vi "Shutdown.vi"(8 "error in (no error)":errorcluster, 9 "Wait Timeout [10000 ms]":i32=10000, 10 "Wait For Shutdown (F)":bool, 11 "Actor API in":refnum<class "Actor API.lvclass">) -> (0 "error out":errorcluster)   [LabVIEW 2015, in "Actor API.lvclass"]
uses:
  Actor API.lvclass
  <vilib>/event_ctls.llb/usereventprio.ctl
  Messaging/Message/Message.lvclass
  Messaging/Message/Message.lvclass/Message.ctl
  Utility/Error Code.ctl
panel:
  # "Note this VI is reentrant as it is called in parallel when shutting down the Top Level"
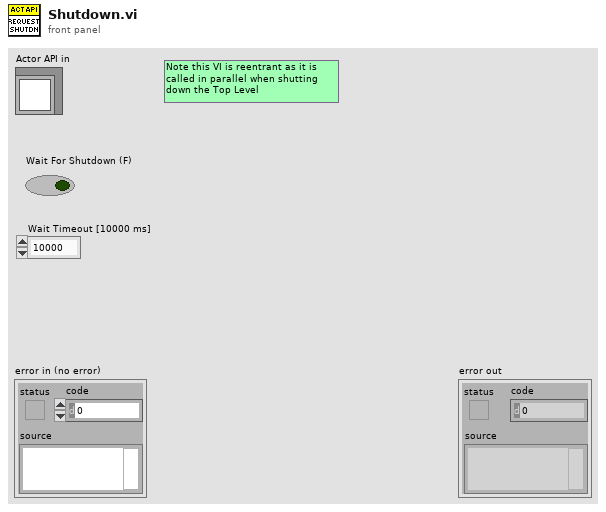
[diagram p1: front panel]
types:
  T1 = typedef "usereventprio.ctl" = enum32{"high priority", "normal priority"}
  T2 = typedef "Error Code.ctl" = enum16{"Actor not found", "Wait for reply timed out", "Framework Error", "Actor not OK", "Error Starting Measurement"}
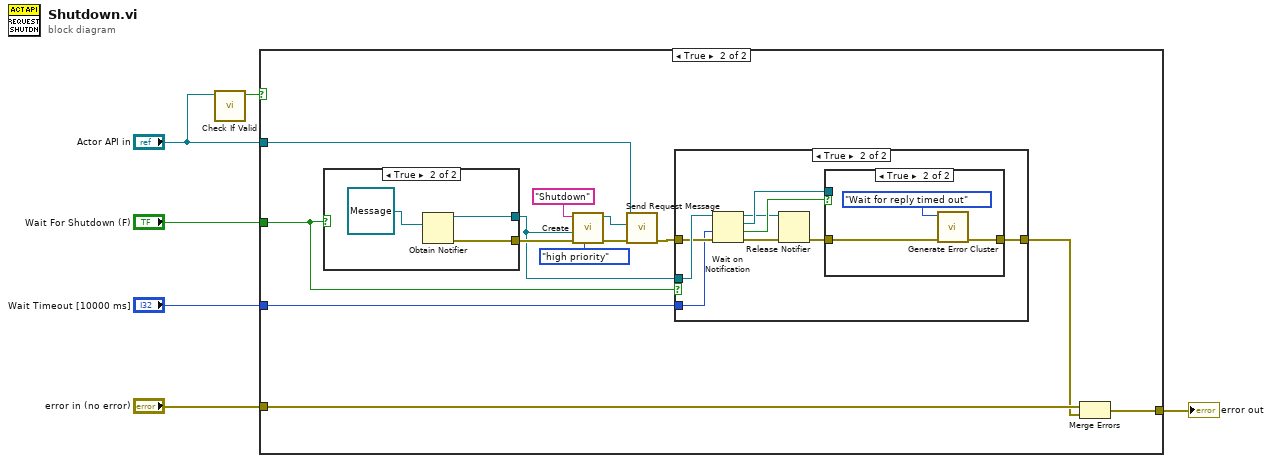
[diagram p0: block diagram]
diagram:
  n1 = call-dynamic "Check If Valid.vi"("Actor API in"="Actor API in") -> ("Valid"=w1:bool)  [unwired: 10 in]
  n2 = case shown="True" w1 {
    tunnel: "Wait Timeout [10000 ms]" -> [_ w20]
    tunnel: "error in (no error)" -> [w7 w12]
    tunnel: [w7 w10] -> w4
    tunnel: "Actor API in" -> [_ w9]
    tunnel: "Wait For Shutdown (F)" -> [_ w8]
    frame False {
    }
    frame True {
      n3 = case shown="True" w8 {
        tunnel: [_ w37] -> w18
        tunnel: [_ w35] -> w17
        frame False {
        }
        frame True {
          n4 = Obtain Notifier(notification data type=refnum<class "Message.lvclass"> refnum ("Message - Actor.lvclass")) -> (notifier out=w35:refnum<notifier>, error out=w37:errorcluster)  [unwired: 3 in, 1 out]
        }
      }
      n5 = call "Create.vi"("Priority (normal)"=usereventprio."high priority", "error in (no error)"=w18, "Reply Channel"=w17, "Name"="Shutdown" ("format string")) -> ("error out"=w19:errorcluster, "Message out"=w14:refnum<class "Message.lvclass">)  [unwired: 6 in]
      n6 = call-dynamic "Send Request Message.vi"("error in (no error)"=w19, "Message"=w14, "Actor API in"=w9) -> ("error out"=w16:errorcluster)  [unwired: 8 in]
      n7 = case shown="True" w8 {
        tunnel: w17 -> [_ w30]
        tunnel: w16 -> [w21 w29]
        tunnel: [w21 w26] -> w11
        tunnel: w20 -> [_ w28]
        frame False {
        }
        frame True {
          n8 = Wait on Notification(notifier=w30, timeout in ms (-1)=w28, error in (no error)=w29) -> (notifier out=w22:refnum<notifier>, notification=w25:refnum<class "Message.lvclass">, timed out?=w27:bool, error out=w24:errorcluster)  [unwired: 1 in]
          n9 = Release Notifier(notifier=w22, error in (no error)=w24) -> (error out=w23:errorcluster)  [unwired: 1 in, 2 out]
          n10 = case shown="True" w27 {
            tunnel: w23 -> [w31 w34]
            tunnel: [w31 w33] -> w26
            tunnel: w25 -> [_ _]
            frame False {
              # "Reply received"
            }
            frame True {
              n11 = call "Generate Error Cluster.vi"("error in (no error)"=w34, "Error"=Error_Code."Wait for reply timed out") -> ("error out"=w33:errorcluster)  [unwired: 9 in]
            }
          }
        }
      }
      n12 = Merge Errors(w12, w11) -> (w10:errorcluster)
    }
  }
  "error out" <- w4
